vi "FindAnnuals.vi"() -> ()   [LabVIEW 2024]
uses:
  db5c1dc2-56b5-4c0d-82d3-cca12777ff98.vi
panel:
  in  "show owning dirs":bool
  in  "search string":string[](array[string])
  in  "Listbox":i32(listbox)
  in  "Path":path
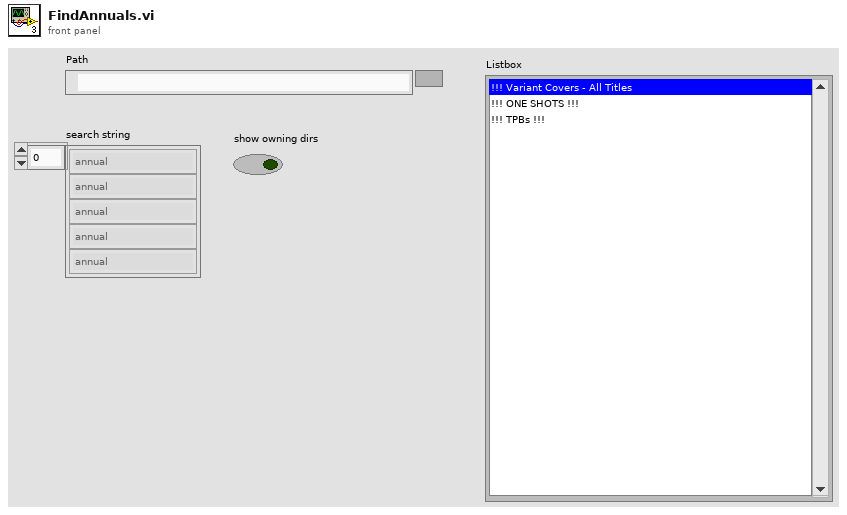
[diagram p1: front panel]
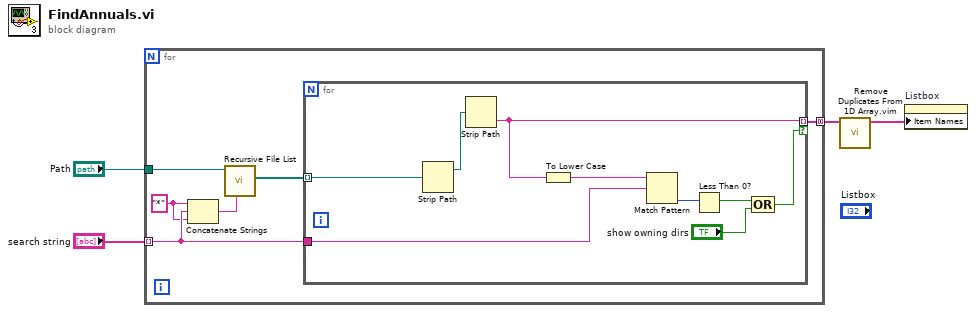
[diagram p0: block diagram]
diagram:
  n1 = for {
    tunnel: "Path" -> [w10]
    tunnel: [w8] -> w3 mode=concatenating
    tunnel: "search string" -> [w6] mode=indexing
    w5 = "*" ("string")
    n2 = Concatenate Strings(w5, w6, w5) -> (w7:string)
    n3 = call <vilib>:"Recursive File List.vi"("pattern"=w7, "Folder Path"=w10) -> ("All Files in Dir"=w9:path[])  [unwired: 5 in, 4 out]
    n4 = for {
      tunnel: w9 -> [w19] mode=indexing
      tunnel: [w14] -> w8 mode=indexing if=w11
      tunnel: w6 -> [w16]
      n5 = Strip Path(path=w19) -> (stripped path=w17:path)  [unwired: 1 out]
      n6 = Strip Path(path=w17) -> (name=w14:string)  [unwired: 1 out]
      n7 = To Lower Case(string=w14) -> (all lower case string=w18:string)
      n8 = Match Pattern(string=w18, regular expression=w16) -> (offset past match=w15:i32)  [unwired: 1 in, 3 out]
      n9 = Less Than 0?(x=w15) -> (x < 0?=w13:bool)
      n10 = Compound Arithmetic op=OR(w13, "show owning dirs") -> (w11:bool)
    }
  }
  n11 = call "Remove Duplicates From 1D Array.vim"("array"=w3) -> ("array with duplicates removed"=w2:string[])  [unwired: 10 in]
  n12 = property on="Listbox" class="LstBox (strict)"("Item Names"=w2) -> ()  [unwired: 2 in, 2 out]
